vi "Result.Numeric, Convert V2 to Measurement V1 Format.vi"(11 "Measurement":T3 {"Status" items=["LOG", "PASS", "FAIL", "ERROR"]}) -> (3 "Meas":T1 {"Status" items=["LOG", "PASS", "FAIL", "ERROR"]})   [LabVIEW 2024]
uses:
  Result.Numeric.ctl
  Result.Limit Type.ctl
  Result.Measurement and Attribute Item Status.ctl
  Result.Measurement Item.ctl
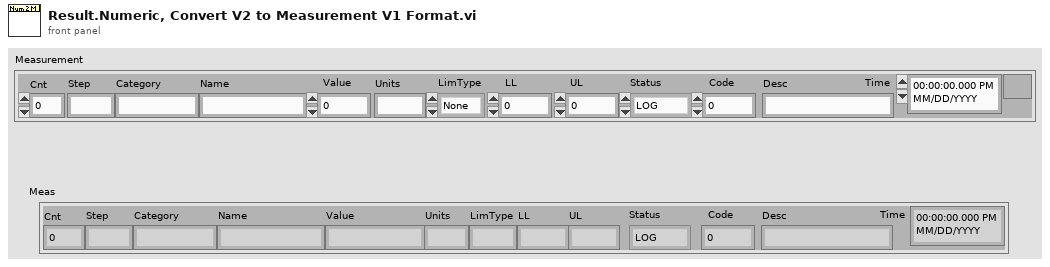
[diagram p1: front panel]
types:
  T1 = typedef "Result.Measurement Item.ctl" = cluster{"Cnt":i32, "Step":string, "Category":string, "Name":string, "Value":string, "Units":string, "LimType":string, "LL":string, "UL":string, "Status":T2, "Code":i32, "Desc":string, "Time":timestamp}
  T2 = typedef "Result.Measurement and Attribute Item Status.ctl" = i32
  T3 = typedef "Result.Numeric.ctl" = cluster{"Cnt":i32, "Step":string, "Category":string, "Name":string, "Value":dbl, "Units":string, "LimType":T4, "LL":dbl, "UL":dbl, "Status":T2, "Code":i32, "Desc":string, "Time":timestamp}
  T4 = typedef "Result.Limit Type.ctl" = enum16{"None", "EQ", "NE", "GT", "LT", "GE", "LE", "GTLT", "GELE", "GELT", "GTLE", "LTGT", "LEGE", "LEGT", "LTGE", "Contains", "NotContains"}
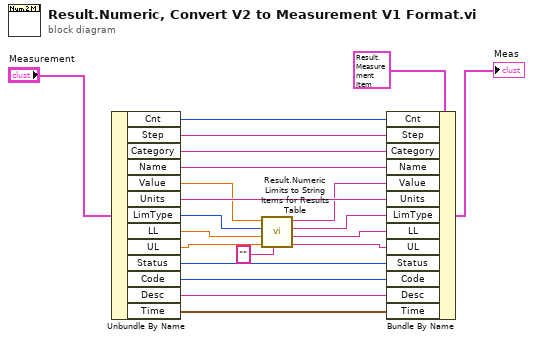
[diagram p0: block diagram]
diagram:
  n1 = Unbundle By Name("Measurement") -> ("Cnt"=w18:i32, "Step"=w17:string, "Category"=w16:string, "Name"=w15:string, "Value"=w9:dbl, "Units"=w10:string, "LimType"=w4:T4, "LL"=w3:dbl, "UL"=w2:dbl, "Status"=w11:T2, "Code"=w14:i32, "Desc"=w13:string, "Time"=w12:timestamp)
  n2 = call "Result.Numeric Limits to String Items for Results Table.vi"("N/A Filler"="", "UL"=w2, "LL"=w3, "LimType"=w4, "Value"=w9) -> ("UL"=w5:string, "LL"=w6:string, "LimType"=w7:string, "Value"=w8:string)  [unwired: 3 in]
  n3 = Bundle By Name(cluster=T1 {"Cnt"=0, "Step"="", "Category"="", "Name"="", "Value"="", "Units"="", "LimType"="", "LL"="", "UL"="", "Status"=0, "Code"=0, "Desc"="", "Time"=timestamp(0 s since 1904-01-01)} ("Meas"), "Cnt"=w18, "Step"=w17, "Category"=w16, "Name"=w15, "Value"=w8, "Units"=w10, "LimType"=w7, "LL"=w6, "UL"=w5, "Status"=w11, "Code"=w14, "Desc"=w13, "Time"=w12) -> (→"Meas":T1)
